vi "Check Serial data.vi"(8 "error in":errorcluster, 11 "Buffer in":string) -> (0 "error out":errorcluster, 2 "Good?":bool, 3 "Buffer out":string)   [LabVIEW 2019, in "PGC2D.lvlib"]
uses:
  PGC2D.lvlib
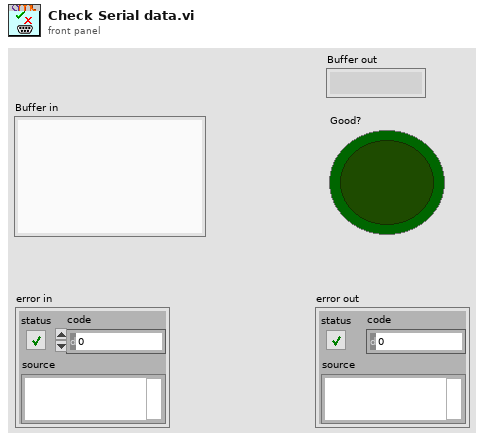
[diagram p1: front panel]
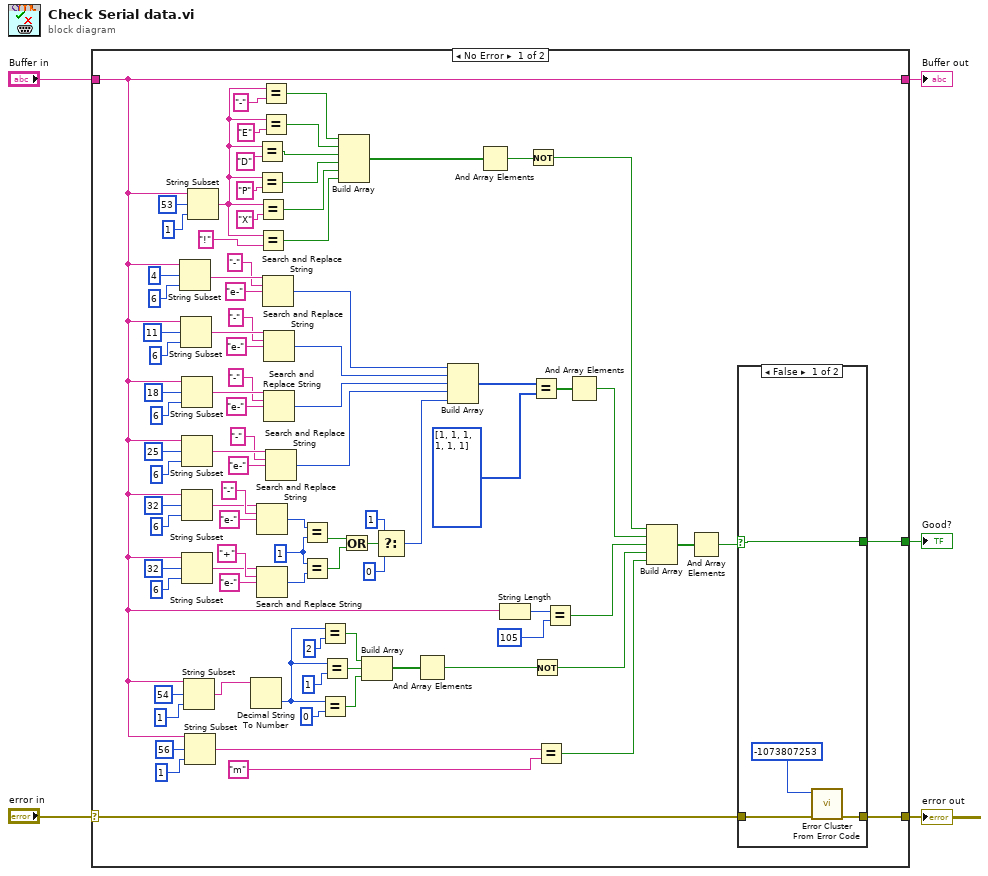
[diagram p0: block diagram]
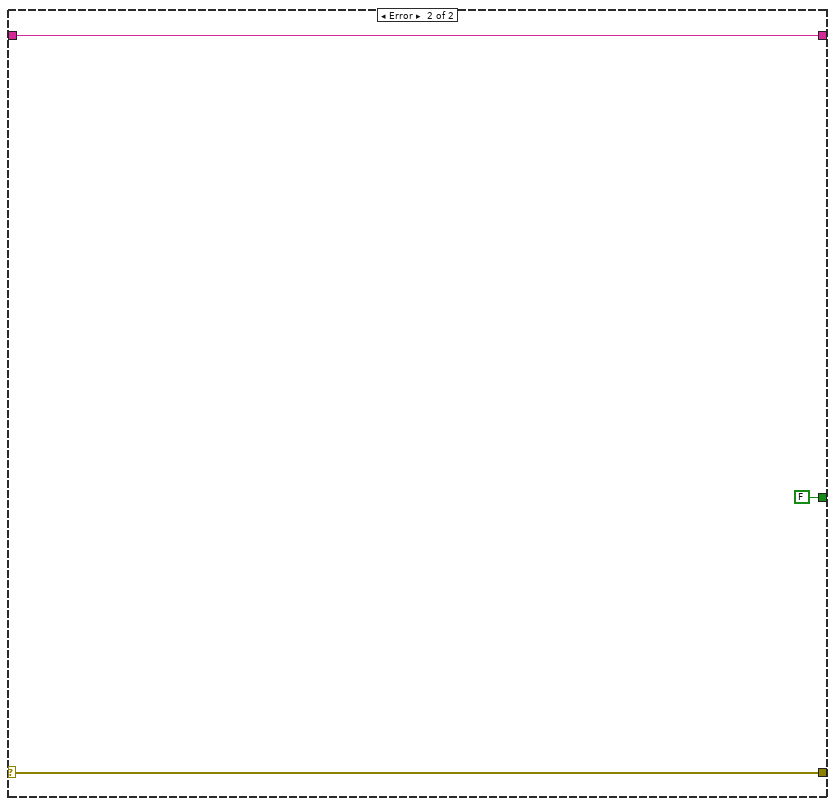
[diagram p3: hidden frame]
diagram:
  n1 = case shown="No Error" "error in" {
    selector: "error in" -> [w25 w106]
    tunnel: "Buffer in" -> [w6 w105]
    tunnel: [w7 w106] -> w3
    tunnel: [w24 FALSE] -> w2
    tunnel: [w6 w105] -> w1
    frame No Error {
      w12 = 1
      n2 = String Subset(string=w6, offset (0)=4, length (rest)=6 ("length (rest)")) -> (substring=w88:string)
      n3 = String Subset(string=w6, offset (0)=11, length (rest)=6 ("length (rest)")) -> (substring=w91:string)
      n4 = String Subset(string=w6, offset (0)=18, length (rest)=6 ("length (rest)")) -> (substring=w94:string)
      n5 = String Subset(string=w6, offset (0)=25, length (rest)=6 ("length (rest)")) -> (substring=w97:string)
      n6 = String Subset(string=w6, offset (0)=32, length (rest)=6 ("length (rest)")) -> (substring=w83:string)
      n7 = String Subset(string=w6, offset (0)=32, length (rest)=6 ("length (rest)")) -> (substring=w16:string)
      n8 = String Subset(string=w6, offset (0)=54, length (rest)=1 ("length (rest)")) -> (substring=w82:string)
      n9 = String Subset(string=w6, offset (0)=56, length (rest)=1 ("length (rest)")) -> (substring=w56:string)
      n10 = String Subset(string=w6, offset (0)=53, length (rest)=1 ("length (rest)")) -> (substring=w45:string)
      n11 = Decimal String To Number(string=w82) -> (number=w54:i32)  [unwired: 2 in, 1 out]
      n12 = Equal?(x=w45, y="D") -> (x = y?=w36:bool)
      n13 = Equal?(x=w45, y="P") -> (x = y?=w35:bool)
      n14 = Search and Replace String(input string=w83, search string="-", replace string="e-" ("replace string (\"\")")) -> (number of replacements=w11:i32)  [unwired: 5 in, 3 out]
      n15 = Search and Replace String(input string=w16, search string="+", replace string="e-" ("replace string (\"\")")) -> (number of replacements=w10:i32)  [unwired: 5 in, 3 out]
      n16 = Equal?(x=w45, y="X") -> (x = y?=w34:bool)
      n17 = Equal?(x=w45, y="!") -> (x = y?=w33:bool)
      n18 = Equal?(x=w45, y="-") -> (x = y?=w38:bool)
      n19 = Equal?(x=w45, y="E") -> (x = y?=w37:bool)
      n20 = Search and Replace String(input string=w88, search string="-", replace string="e-" ("replace string (\"\")")) -> (number of replacements=w65:i32)  [unwired: 5 in, 3 out]
      n21 = Search and Replace String(input string=w91, search string="-", replace string="e-" ("replace string (\"\")")) -> (number of replacements=w62:i32)  [unwired: 5 in, 3 out]
      n22 = Search and Replace String(input string=w94, search string="-", replace string="e-" ("replace string (\"\")")) -> (number of replacements=w63:i32)  [unwired: 5 in, 3 out]
      n23 = Search and Replace String(input string=w97, search string="-", replace string="e-" ("replace string (\"\")")) -> (number of replacements=w64:i32)  [unwired: 5 in, 3 out]
      n24 = Equal?(x=w11, y=w12) -> (x = y?=w9:bool)
      n25 = Equal?(x=w12, y=w10) -> (x = y?=w8:bool)
      n26 = Equal?(x=w54, y=2) -> (x = y?=w48:bool)
      n27 = Equal?(x=w54, y=0) -> (x = y?=w50:bool)
      n28 = Equal?(x=w54, y=1) -> (x = y?=w49:bool)
      n29 = Build Array(w38, w37, w36, w35, w34, w33) -> (w32:bool[])
      n30 = Or(x=w9, y=w8) -> (x .or. y?=w13:bool)
      n31 = Build Array(w48, w49, w50) -> (w47:bool[])
      n32 = Select(t=1, s=w13, f=0) -> (s? t:f=w20:i32)
      n33 = And Array Elements(Boolean array=w47) -> (logical AND=w46:bool)
      n34 = Build Array(w65, w62, w63, w64, w20) -> (w61:i32[])
      n35 = And Array Elements(Boolean array=w32) -> (logical AND=w23:bool)
      n36 = String Length(string=w6) -> (length=w58:i32)
      n37 = Not(x=w23) -> (.not. x?=w22:bool)
      n38 = Equal?(x=w61, y=i32[] [1, 1, 1, 1, 1, 1]) -> (x = y?=w60:bool[])
      n39 = Not(x=w46) -> (.not. x?=w31:bool)
      n40 = Equal?(x=w56, y="m") -> (x = y?=w30:bool)
      n41 = Equal?(x=w58, y=105) -> (x = y?=w29:bool)
      n42 = And Array Elements(Boolean array=w60) -> (logical AND=w28:bool)
      n43 = Build Array(w22, w28, w29, w31, w30) -> (w27:bool[])
      n44 = And Array Elements(Boolean array=w27) -> (logical AND=w26:bool)
      n45 = case shown="False" w26 {
        selector: w26 -> [w101 w103]
        tunnel: [w98 w102] -> w7
        tunnel: w25 -> [w99 w102]
        tunnel: [w101 w103] -> w24
        frame False {
          n46 = call <vilib>:"Error Cluster From Error Code.vi"("error in (no error)"=w99, "error code (0)"=-1073807253 ("specific error code to clear (0: all)")) -> ("error out"=w98:errorcluster)  [unwired: 7 in]
        }
        frame True {
        }
      }
    }
    frame Error {
    }
  }
  "error out" <- w3
  "Good?" <- w2
  "Buffer out" <- w1
